vi "cRIO.vi"   [LabVIEW 2014]
uses:
  <vilib>/Platform/TimedLoop/XDataNode/timing_clust.ctl
  <vilib>/Platform/TimedLoop/XDataNode/nitl_modes.ctl
  <vilib>/Platform/TimedLoop/XDataNode/wakeup.ctl
  <vilib>/platform/TimedLoop/XDataNode/XDataNode.xnode
  <vilib>/Platform/TimedLoop/XDataNode/XDNodeRunTimeDep.lvlib
types:
  T1 = typedef "XDNodeRunTimeDep.lvlib/timing_clust.ctl" = cluster{"Expected End [f-1]":u64, "Actual End [f-1]":u64, "Finished Late? [f-1]":bool, "Expected End [i-1]":u64, "Actual End [i-1]":u64, "Finished Late? [i-1]":bool, "Expected Start [i]":u64, "Actual Start [i]":u64, "Expected Start [f]":u64, "Actual Start [f]":u64, "Source Name":string, "Structure Name":string, "Period":i64, "Deadline":i64, "Offset":i64, "Start":i64, "Priority":i32, "Timeout":i32, "Mode":T2, "Wakeup Reason":T3, "Error":errorcluster, "Source Type":string, "Secondary Source Type":string, "Global End Time":u64, "Global Start Time":u64, "Frame Duration":u64, "Iteration Duration":u64, "Assigned CPU":i32, "I/O Scan Engine Mode":u32}
  T2 = typedef "XDNodeRunTimeDep.lvlib/nitl_modes.ctl" = enum32{"No Change", "Process missed periods, maintain original phase", "Discard missed periods, maintain original phase", "Process missed periods, ignore original phase", "Discard missed periods, ignore original phase"}
  T3 = typedef "XDNodeRunTimeDep.lvlib/wakeup.ctl" = enum32{"Normal", "Aborted", "Asynchronous wakeup", "Timing source error", "Timed loop error", "Timeout"}
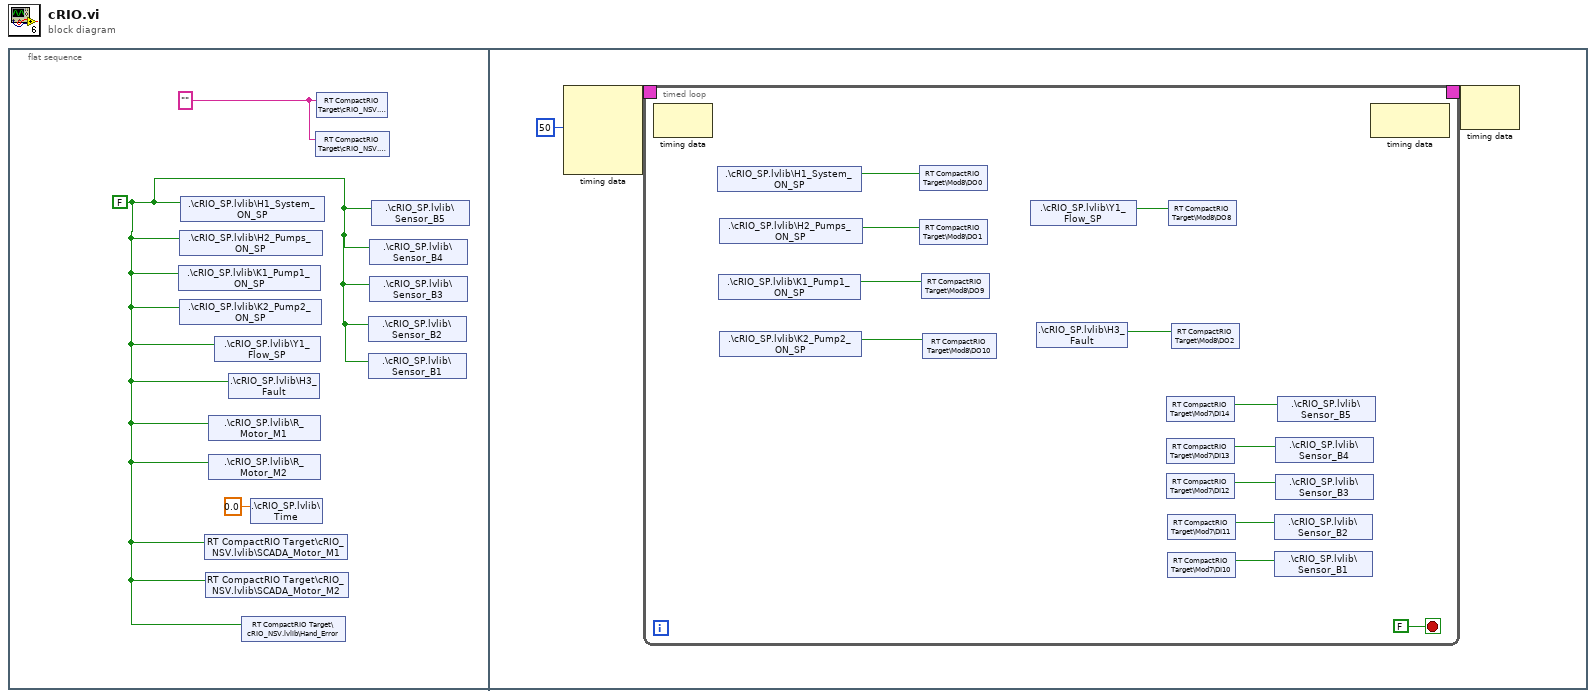
[diagram p0: block diagram]
diagram:
  n1 = flat-sequence {
    frame #0 {
      w3 = ""
      w1 = FALSE
      n2 = shared-variable ".\\cRIO_SP.lvlib\\K1_Pump1_ON_SP"(w1) -> ()  [unwired: 1 in, 1 out]
      n3 = shared-variable ".\\cRIO_SP.lvlib\\H2_Pumps_ON_SP"(w1) -> ()  [unwired: 1 in, 1 out]
      n4 = shared-variable ".\\cRIO_SP.lvlib\\K2_Pump2_ON_SP"(w1) -> ()  [unwired: 1 in, 1 out]
      n5 = shared-variable ".\\cRIO_SP.lvlib\\H1_System_ON_SP"(w1) -> ()  [unwired: 1 in, 1 out]
      n6 = shared-variable "RT CompactRIO Target\\cRIO_NSV.lvlib\\SCADA_Motor_M1"(w1) -> ()  [unwired: 1 in, 1 out]
      n7 = shared-variable "RT CompactRIO Target\\cRIO_NSV.lvlib\\SCADA_Motor_M2"(w1) -> ()  [unwired: 1 in, 1 out]
      n8 = shared-variable ".\\cRIO_SP.lvlib\\R_Motor_M1"(w1) -> ()  [unwired: 1 in, 1 out]
      n9 = shared-variable ".\\cRIO_SP.lvlib\\R_Motor_M2"(w1) -> ()  [unwired: 1 in, 1 out]
      n10 = shared-variable ".\\cRIO_SP.lvlib\\Y1_Flow_SP"(w1) -> ()  [unwired: 1 in, 1 out]
      n11 = shared-variable ".\\cRIO_SP.lvlib\\H3_Fault"(w1) -> ()  [unwired: 1 in, 1 out]
      n12 = shared-variable "RT CompactRIO Target\\cRIO_NSV.lvlib\\Hand_Error"(w1) -> ()  [unwired: 1 in, 1 out]
      n13 = shared-variable ".\\cRIO_SP.lvlib\\Time"(0.0 ("Time")) -> ()  [unwired: 1 in, 1 out]
      n14 = shared-variable "RT CompactRIO Target\\cRIO_NSV.lvlib\\Tasks"(w3) -> ()  [unwired: 1 in, 1 out]
      n15 = shared-variable "RT CompactRIO Target\\cRIO_NSV.lvlib\\State"(w3) -> ()  [unwired: 1 in, 1 out]
      n16 = shared-variable ".\\cRIO_SP.lvlib\\Sensor_B2"(w1) -> ()  [unwired: 1 in, 1 out]
      n17 = shared-variable ".\\cRIO_SP.lvlib\\Sensor_B1"(w1) -> ()  [unwired: 1 in, 1 out]
      n18 = shared-variable ".\\cRIO_SP.lvlib\\Sensor_B4"(w1) -> ()  [unwired: 1 in, 1 out]
      n19 = shared-variable ".\\cRIO_SP.lvlib\\Sensor_B3"(w1) -> ()  [unwired: 1 in, 1 out]
      n20 = shared-variable ".\\cRIO_SP.lvlib\\Sensor_B5"(w1) -> ()  [unwired: 1 in, 1 out]
    }
    frame #1 {
      n21 = node-c288(i64 50 ("Period")) -> (w6:T1)  [unwired: 3 in]
      n22 = timed-loop {
        timing: w6 -> [_]
        timing-out: [_] -> w5
        stop <- FALSE stop-if-true
        n23 = node-c288() -> ()  [unwired: 1 in, 1 out]
        n24 = shared-variable ".\\cRIO_SP.lvlib\\H1_System_ON_SP"() -> (w18:bool)  [unwired: 1 in, 1 out]
        n25 = shared-variable ".\\cRIO_SP.lvlib\\K1_Pump1_ON_SP"() -> (w12:bool)  [unwired: 1 in, 1 out]
        n26 = shared-variable ".\\cRIO_SP.lvlib\\H2_Pumps_ON_SP"() -> (w17:bool)  [unwired: 1 in, 1 out]
        n27 = shared-variable ".\\cRIO_SP.lvlib\\K2_Pump2_ON_SP"() -> (w13:bool)  [unwired: 1 in, 1 out]
        n28 = shared-variable "RT CompactRIO Target\\Mod8\\DO0"(w18) -> ()  [unwired: 1 in, 1 out]
        n29 = shared-variable "RT CompactRIO Target\\Mod8\\DO1"(w17) -> ()  [unwired: 1 in, 1 out]
        n30 = shared-variable "RT CompactRIO Target\\Mod8\\DO9"(w12) -> ()  [unwired: 1 in, 1 out]
        n31 = shared-variable "RT CompactRIO Target\\Mod8\\DO10"(w13) -> ()  [unwired: 1 in, 1 out]
        n32 = shared-variable ".\\cRIO_SP.lvlib\\Y1_Flow_SP"() -> (w15:bool)  [unwired: 1 in, 1 out]
        n33 = shared-variable ".\\cRIO_SP.lvlib\\H3_Fault"() -> (w14:bool)  [unwired: 1 in, 1 out]
        n34 = shared-variable "RT CompactRIO Target\\Mod7\\DI14"() -> (w11:bool)  [unwired: 1 in, 1 out]
        n35 = shared-variable "RT CompactRIO Target\\Mod7\\DI13"() -> (w10:bool)  [unwired: 1 in, 1 out]
        n36 = shared-variable "RT CompactRIO Target\\Mod7\\DI12"() -> (w9:bool)  [unwired: 1 in, 1 out]
        n37 = shared-variable "RT CompactRIO Target\\Mod7\\DI11"() -> (w8:bool)  [unwired: 1 in, 1 out]
        n38 = shared-variable "RT CompactRIO Target\\Mod7\\DI10"() -> (w7:bool)  [unwired: 1 in, 1 out]
        n39 = shared-variable "RT CompactRIO Target\\Mod8\\DO8"(w15) -> ()  [unwired: 1 in, 1 out]
        n40 = shared-variable "RT CompactRIO Target\\Mod8\\DO2"(w14) -> ()  [unwired: 1 in, 1 out]
        n41 = shared-variable ".\\cRIO_SP.lvlib\\Sensor_B2"(w8) -> ()  [unwired: 1 in, 1 out]
        n42 = shared-variable ".\\cRIO_SP.lvlib\\Sensor_B1"(w7) -> ()  [unwired: 1 in, 1 out]
        n43 = shared-variable ".\\cRIO_SP.lvlib\\Sensor_B4"(w10) -> ()  [unwired: 1 in, 1 out]
        n44 = shared-variable ".\\cRIO_SP.lvlib\\Sensor_B3"(w9) -> ()  [unwired: 1 in, 1 out]
        n45 = shared-variable ".\\cRIO_SP.lvlib\\Sensor_B5"(w11) -> ()  [unwired: 1 in, 1 out]
        n46 = node-c288() -> ()  [unwired: 1 in, 1 out]
      }
      n47 = node-c288(w5) -> ()  [unwired: 1 out]
    }
  }
